vi "FilterChannels.vi"(8 "error in (no error)":errorcluster, 11 "channels":T1[](array[typedef])) -> (0 "error out":errorcluster, 3 "single point channels":T1[](array[typedef]))   [LabVIEW 2017, in "ScanEngine.lvlib"]
uses:
  <vilib>/addons/InsightCM/Devices/Shared/Common/ScanEngine/ScanEngine.lvlib
  <vilib>/addons/InsightCM/MessageBus/Base/controls/R2_Channel.ctl
  <vilib>/addons/InsightCM/MessageBus/Base/controls/KeyValuePair.ctl
  <vilib>/addons/InsightCM/MessageBus/Base/controls/Metric.ctl
  <vilib>/addons/InsightCM/Utilities/PropertyHelpers/PropertyHelpers.lvlib
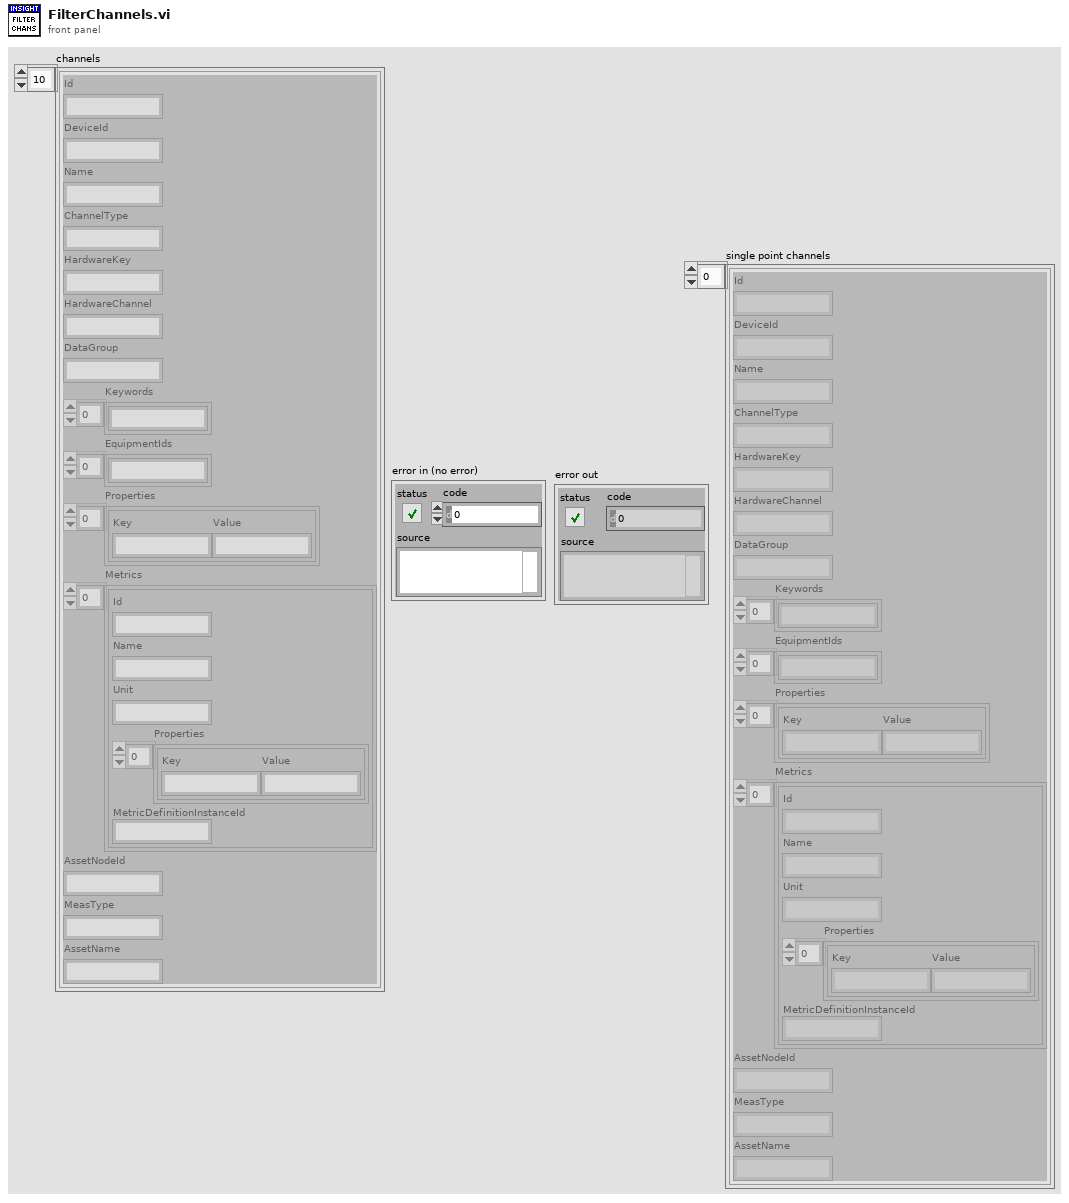
[diagram p1: front panel]
types:
  T1 = typedef "R2_Channel.ctl" = cluster{"Id":string, "DeviceId":string, "Name":string, "ChannelType":string, "HardwareKey":string, "HardwareChannel":string, "DataGroup":string, "Keywords":string[], "EquipmentIds":string[], "Properties":T2[], "Metrics":T3[], "AssetNodeId":string, "MeasType":string, "AssetName":string}
  T2 = typedef "KeyValuePair.ctl" = cluster{"Key":string, "Value":string}
  T3 = typedef "Metric.ctl" = cluster{"Id":string, "Name":string, "Unit":string, "Properties":T2[], "MetricDefinitionInstanceId":string}
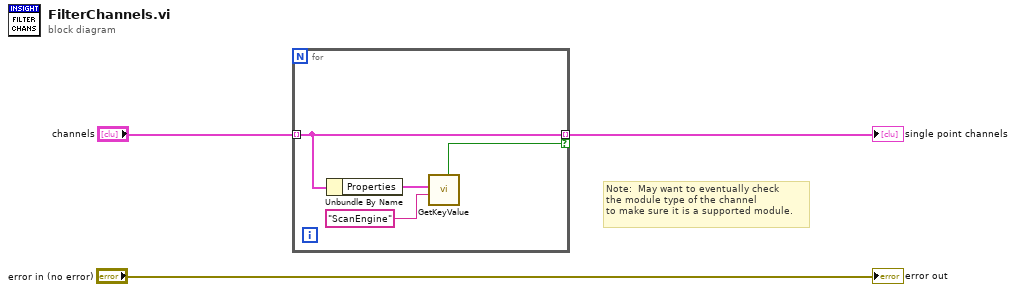
[diagram p0: block diagram]
diagram:
  # "Note:  May want to eventually check\nthe module type of the channel\nto make sure it is a supported module."
  n1 = for {
    tunnel: "channels" -> [w5] mode=indexing
    tunnel: [w5] -> w2 mode=indexing if=w4
    n2 = Unbundle By Name(w5) -> ("Properties"=w7:T2[])
    n3 = call <vilib>:"GetKeyValue.vi"("key"="ScanEngine" ("name"), "key value pairs"=w7) -> ("found"=w4:bool)  [unwired: 7 in, 2 out]
  }
  "single point channels" <- w2
  "error out" <- "error in (no error)"
